vi "Read Configuration.vi"(8 "error in (no error)":errorcluster, 11 "文件名":string="myDAQConfi.ini") -> (0 "error out":errorcluster, 3 "Configuration":T1={"DAQmxChannel myVolt"={"DAQmxChannel myVinput1"={"PhysicalChanName"="", "AI_Voltage_Units"=10348, "AI_Max"=5.0, "AI_Min"=-5.0}, "DAQmxChannel myVinput2"={"PhysicalChanName"="", "AI_Voltage_Units"=10348, "AI_Max"=5.0, "AI_Min"=-5.0}, "DAQmxChannel myVoutput1"={"PhysicalChanName"="", "AI_Min"=-5.0, "AI_Max"=5.0, "AI_Voltage_Units"=10348}, "DAQmxChannel myVoutput2"={"PhysicalChanName"="", "AI_Min"=-5.0, "AI_Max"=5.0, "AI_Voltage_Units"=10348}, "Saidmple Clock Input"={"rate"=1000.0, "samples per channel"=100}, "Saidmple Clock Output"={"rate"=1000.0, "samples per channel"=100}}, "Dev"=""} {"DAQmxChannel myVolt"."DAQmxChannel myVoutput2"."AI_Voltage_Units" items=["伏特"=10348, "来自自定义换算"=10065]; "DAQmxChannel myVolt"."DAQmxChannel myVoutput1"."AI_Voltage_Units" items=["伏特"=10348, "来自自定义换算"=10065]; "DAQmxChannel myVolt"."DAQmxChannel myVinput1"."AI_Voltage_Units" items=["伏特"=10348, "来自自定义换算"=10065]; "DAQmxChannel myVolt"."DAQmxChannel myVinput2"."AI_Voltage_Units" items=["伏特"=10348, "来自自定义换算"=10065]})   [LabVIEW 2016]
uses:
  Contral/Coniguration.ctl
  <vilib>/NI/GXML/_subVIs/GXML SearchParser/Search Parser.vi
  <vilib>/NI/GXML/GXML.lvlib
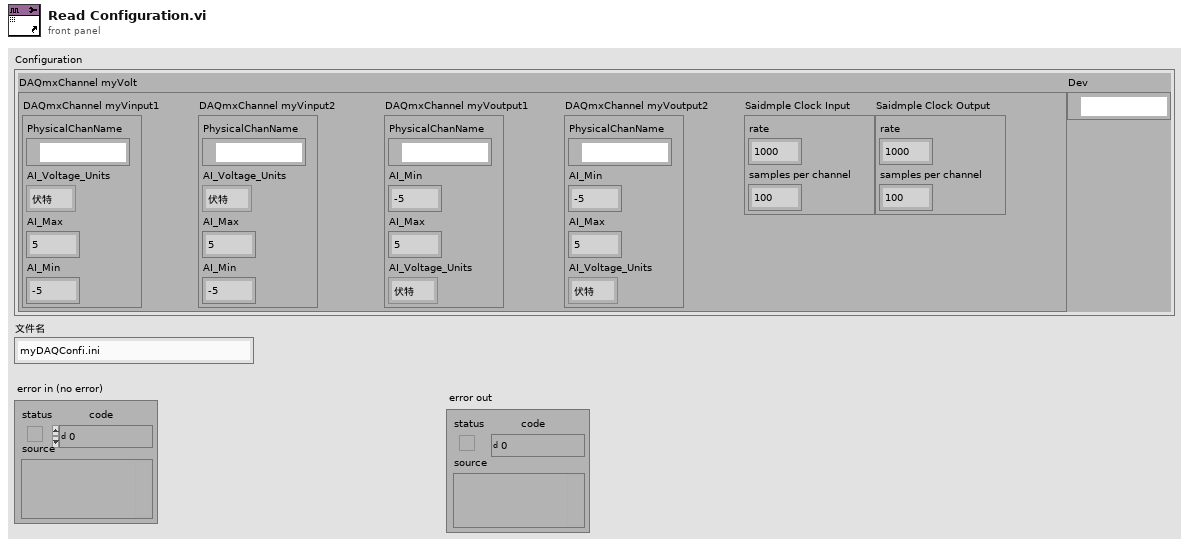
[diagram p1: front panel]
types:
  T1 = typedef "Coniguration.ctl" = cluster{"DAQmxChannel myVolt":cluster{"DAQmxChannel myVinput1":cluster{"PhysicalChanName":tag, "AI_Voltage_Units":i32, "AI_Max":dbl, "AI_Min":dbl}, "DAQmxChannel myVinput2":cluster{"PhysicalChanName":tag, "AI_Voltage_Units":i32, "AI_Max":dbl, "AI_Min":dbl}, "DAQmxChannel myVoutput1":cluster{"PhysicalChanName":tag, "AI_Min":dbl, "AI_Max":dbl, "AI_Voltage_Units":i32}, "DAQmxChannel myVoutput2":cluster{"PhysicalChanName":tag, "AI_Min":dbl, "AI_Max":dbl, "AI_Voltage_Units":i32}, "Saidmple Clock Input":cluster{"rate":dbl, "samples per channel":i32}, "Saidmple Clock Output":cluster{"rate":dbl, "samples per channel":i32}}, "Dev":tag}
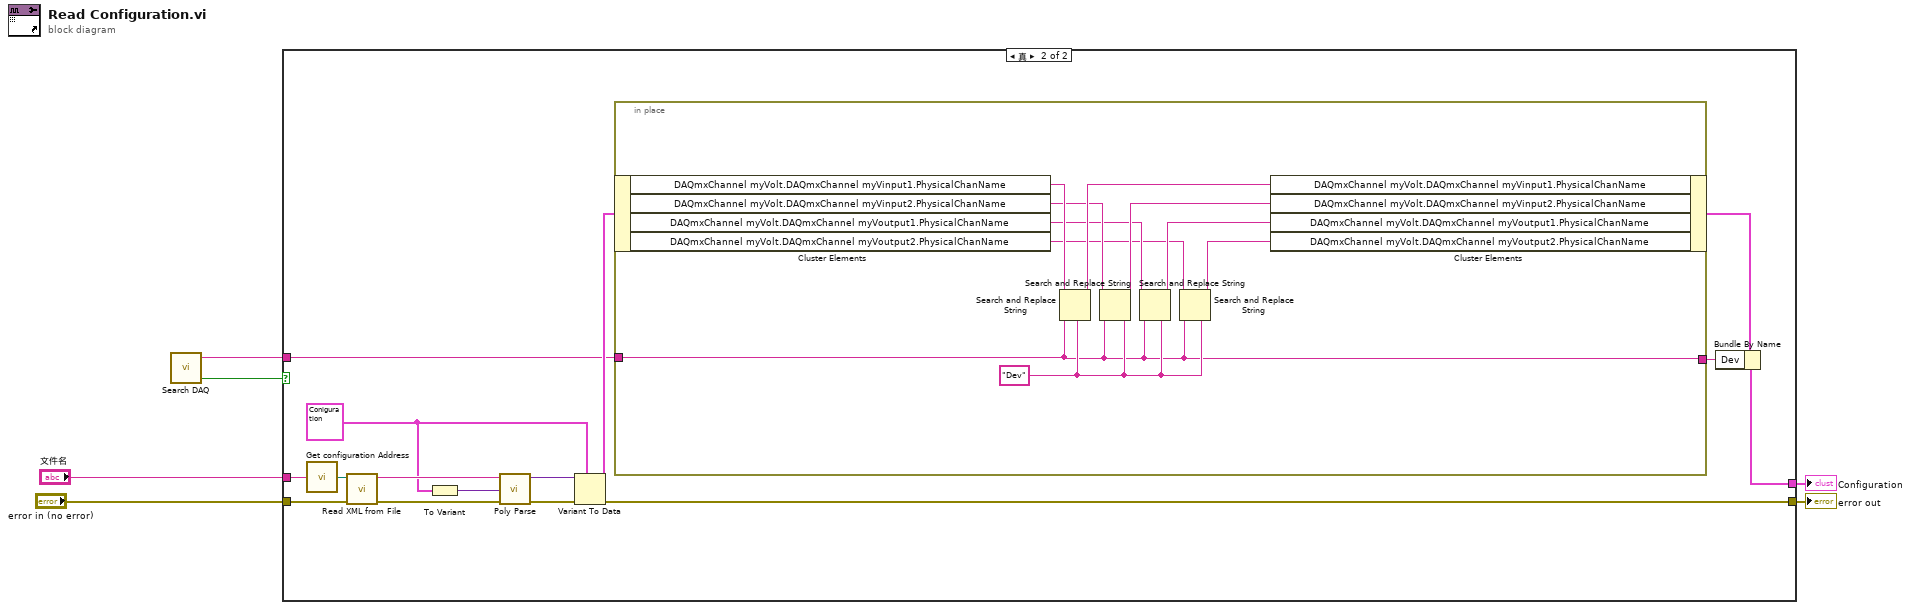
[diagram p0: block diagram]
diagram:
  n1 = call "Search DAQ.vi"() -> ("Dev"=w3:tag, "仪器是否存在？"=w1:bool)  [unwired: 8 in]
  n2 = case shown="真" w1 {
    tunnel: "文件名" -> [_ w22]
    tunnel: "error in (no error)" -> [w7 w21]
    tunnel: [w7 w20] -> w4
    tunnel: w3 -> [_ w11]
    tunnel: [_ w8] -> w2
    frame False {
    }
    frame True {
      w15 = T1 {"DAQmxChannel myVolt"={"DAQmxChannel myVinput1"={"PhysicalChanName"="", "AI_Voltage_Units"=0, "AI_Max"=0.0, "AI_Min"=0.0}, "DAQmxChannel myVinput2"={"PhysicalChanName"="", "AI_Voltage_Units"=0, "AI_Max"=0.0, "AI_Min"=0.0}, "DAQmxChannel myVoutput1"={"PhysicalChanName"="", "AI_Min"=0.0, "AI_Max"=0.0, "AI_Voltage_Units"=0}, "DAQmxChannel myVoutput2"={"PhysicalChanName"="", "AI_Min"=0.0, "AI_Max"=0.0, "AI_Voltage_Units"=0}, "Saidmple Clock Input"={"rate"=1000.0, "samples per channel"=100}, "Saidmple Clock Output"={"rate"=1000.0, "samples per channel"=100}}, "Dev"="myDAQ2"} ("Configuration")
      n3 = call "Get configuration Address.vi"("文件名"=w22) -> ("配置文件路径"=w19:path)
      n4 = call <vilib>:"Read XML from File.vi"("error in"=w21, "XML File Path"=w19) -> ("error out"=w14:errorcluster, "XML String Out"=w18:string)  [unwired: 8 in]
      n5 = To Variant(anything=w15) -> (Variant=w17:variant)
      n6 = call-poly <vilib>:"Poly Parse.vi"("error in"=w14, "TypeDesc"=w17, "XML String In"=w18) -> ("error out"=w13:errorcluster, "Parsed Data"=w16:variant)  [unwired: 7 in]
      n7 = Variant To Data(error in=w13, type=w15, Variant=w16) -> (data=w12:T1, error out=w20:errorcluster)
      n8 = in-place {
        in-place-border: w11 -> [w23]
        in-place-border: [w23] -> w10
        w30 = "Dev" ("搜索字符串")
        n9 = in-place-cluster #1(w12) -> ("DAQmxChannel myVolt.DAQmxChannel myVinput1.PhysicalChanName"=w32:tag, "DAQmxChannel myVolt.DAQmxChannel myVinput2.PhysicalChanName"=w29:tag, "DAQmxChannel myVolt.DAQmxChannel myVoutput1.PhysicalChanName"=w27:tag, "DAQmxChannel myVolt.DAQmxChannel myVoutput2.PhysicalChanName"=w25:tag)
        n10 = Search and Replace String(input string=w32, search string=w30, replace string=w23) -> (result string=w31:string)  [unwired: 5 in, 3 out]
        n11 = Search and Replace String(input string=w29, search string=w30, replace string=w23) -> (result string=w28:string)  [unwired: 5 in, 3 out]
        n12 = Search and Replace String(input string=w27, search string=w30, replace string=w23) -> (result string=w26:string)  [unwired: 5 in, 3 out]
        n13 = Search and Replace String(input string=w25, search string=w23, replace string=w30) -> (result string=w24:string)  [unwired: 5 in, 3 out]
        n14 = in-place-cluster #1("DAQmxChannel myVolt.DAQmxChannel myVinput1.PhysicalChanName"=w31, "DAQmxChannel myVolt.DAQmxChannel myVinput2.PhysicalChanName"=w28, "DAQmxChannel myVolt.DAQmxChannel myVoutput1.PhysicalChanName"=w26, "DAQmxChannel myVolt.DAQmxChannel myVoutput2.PhysicalChanName"=w24) -> (w9:T1)
      }
      n15 = Bundle By Name(cluster=w9, "Dev"=w10) -> (w8:T1)
    }
  }
  "error out" <- w4
  "Configuration" <- w2
